vi "TankDrive.vi"   [LabVIEW 2011]
uses:
  <vilib>/Rock Robotics/WPI/Solenoid/Deprecated/WPI_SolenoidSetBool.vi
types:
  T1 = typedef "WPI_SolenoidDevRef.ctl" = cluster{"DevStatus":errorcluster, "Solenoid Module":T2, "Forward Solenoid Channel":T3, "Reverse Solenoid Channel":T3}
  T2 = typedef "FPGA_TypedefSolenoidModule.ctl" = enum16{"Solenoid Module 1", "Solenoid Module 2"}
  T3 = typedef "WPI_SolenoidChannel.ctl" = enum8{"Solenoid 1", "Solenoid 2", "Solenoid 3", "Solenoid 4", "Solenoid 5", "Solenoid 6", "Solenoid 7", "Solenoid 8", "Invalid"}
  T4 = typedef "WPI_JoystickDevRef.ctl" = cluster{"Device":T5}
  T5 = typedef "WPI_JoystickDeviceEnum.ctl" = enum16{"USB 1", "USB 2", "USB 3", "USB 4", "Kinect 1", "Kinect 2"}
  T6 = typedef "WPI_RobotDriveDevRef.ctl" = cluster{"DevStatus":errorcluster, "Motors[]":T7[], "Square Inputs":bool, "Max Output":dbl, "Isochronous":bool}
  T7 = typedef "WPI_MotorControlDeviceRef.ctl" = cluster{"DeviceStatus":errorcluster, "Type":enum16{"PWM", "CAN"}, "PWM":cluster{"Digital Module":T8, "PWM Channel":T9, "DeadBand":T10}, "CAN":cluster{"Device Number":u8, "Control Mode":T11, "Semaphore":T12, "Max Vout":dbl}, "Invert":bool, "TransformRef":T13, "InvTransformRef":T13}
  T8 = typedef "FPGA_TypedefDigitalModule.ctl" = enum16{"Digital Module 1", "Digital Module 2"}
  T9 = typedef "FPGA_DIOPWMChannel.ctl" = enum8{"PWM 1", "PWM 2", "PWM 3", "PWM 4", "PWM 5", "PWM 6", "PWM 7", "PWM 8", "PWM 9", "PWM 10", "Invalid"}
  T10 = typedef "WPI_PWMDeadband.ctl" = cluster{"Name":string, "maxPositivePwm":i32, "minPositivePwm":i32, "centerPwm":i32, "maxNegativePwm":i32, "minNegativePwm":i32, "angularRange":u16}
  T11 = typedef "WPI_CANJaguar_ControlMode.ctl" = enum8{"Percent VBus", "Current", "Speed", "Position", "Voltage"}
  T12 = typedef "Semaphore RefNum" = refnum<k1>
  T13 = typedef "WPI_PWMTransform_ConPane.ctl" = refnum<vi>
  T14 = typedef "WPI_JoystickButtonState.ctl" = cluster{"Button 1":bool, "Button 2":bool, "Button 3":bool, "Button 4":bool, "Button 5":bool, "Button 6":bool, "Button 7":bool, "Button 8":bool, "Button 9":bool, "Button 10":bool, "Button 11":bool, "Button 12":bool}
  T15 = cluster{"axis 1 (x)":dbl, "axis 2 (y)":dbl, "axis 3 (throttle)":dbl, "axis 4":dbl, "axis 5":dbl, "axis 6":dbl}
  T16 = typedef "WPI_DigitalOutputDevRef.ctl" = cluster{"Digital Module":T8, "DIO Channel":T17, "DevStatus":errorcluster}
  T17 = typedef "FPGA_DIOChannel.ctl" = enum8{"DIO 1", "DIO 2", "DIO 3", "DIO 4", "DIO 5", "DIO 6", "DIO 7", "DIO 8", "DIO 9", "DIO 10", "DIO 11", "DIO 12", "DIO 13", "DIO 14", "Invalid"}
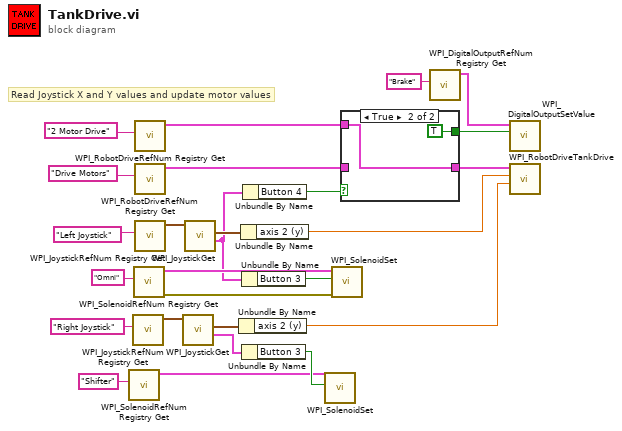
[diagram p0: block diagram]
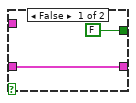
[diagram p2: hidden frame]
diagram:
  # "Read Joystick X and Y values and update motor values"
  n1 = call <vilib>:"WPI_SolenoidRefNum Registry Get.vi"("refnum name"="Shifter") -> ("SolenoidDevRef"=w24:T1)  [unwired: 1 in, 9 out]
  n2 = call <vilib>:"WPI_JoystickRefNum Registry Get.vi"("refnum name"="Right Joystick") -> ("JoystickDevRef"=w21:T4)  [unwired: 1 in, 9 out]
  n3 = call <vilib>:"WPI_SolenoidRefNum Registry Get.vi"("refnum name"="Omni") -> ("error out"=w11:errorcluster, "SolenoidDevRef"=w12:T1)  [unwired: 9 in]
  n4 = call <vilib>:"WPI_RobotDriveRefNum Registry Get.vi"("refnum name"="2 Motor Drive") -> ("RobotDriveDevRef"=w7:T6)  [unwired: 1 in, 9 out]
  n5 = call <vilib>:"WPI_RobotDriveRefNum Registry Get.vi"("refnum name"="Drive Motors") -> ("RobotDriveDevRef"=w4:T6)  [unwired: 1 in, 9 out]
  n6 = call <vilib>:"WPI_JoystickRefNum Registry Get.vi"("refnum name"="Left Joystick") -> ("JoystickDevRef"=w18:T4)  [unwired: 1 in, 9 out]
  n7 = call <vilib>:"WPI_JoystickGet.vi"("JoystickDevRef"=w21) -> ("Buttons"=w23:T14, "Axes"=w19:T15)  [unwired: 1 in, 4 out]
  n8 = call <vilib>:"WPI_JoystickGet.vi"("JoystickDevRef"=w18) -> ("Buttons"=w8:T14, "Axes"=w16:T15)  [unwired: 1 in, 4 out]
  n9 = Unbundle By Name(w19) -> ("axis 2 (y)"=w22:dbl)
  n10 = Unbundle By Name(w16) -> ("axis 2 (y)"=w15:dbl)
  n11 = Unbundle By Name(w8) -> ("Button 3"=w10:bool)
  n12 = Unbundle By Name(w23) -> ("Button 3"=w26:bool)
  n13 = Unbundle By Name(w8) -> ("Button 4"=w5:bool)
  n14 = call-poly <vilib>:"WPI_SolenoidSet.vi"("Value"=w26, "SolenoidDevRef"=w24) -> ()  [unwired: 1 in, 9 out]
  n15 = call-poly <vilib>:"WPI_SolenoidSet.vi"("error in (no error)"=w11, "Value"=w10, "SolenoidDevRef"=w12) -> ()  [unwired: 7 in, 2 out]
  n16 = case shown="True" w5 {
    tunnel: w7 -> [_ w30]
    tunnel: [w28 w30] -> w6
    tunnel: w4 -> [w28 _]
    tunnel: [FALSE ("Value") TRUE ("Value")] -> w1
    frame False {
    }
    frame True {
    }
  }
  n17 = call <vilib>:"WPI_DigitalOutputRefNum Registry Get.vi"("refnum name"="Brake") -> ("DigitalOutputDevRef"=w2:T16)  [unwired: 9 in, 1 out]
  n18 = call <vilib>:"WPI_DigitalOutputSetValue.vi"("Value"=w1, "DigitalOutputDevRef"=w2) -> ()  [unwired: 8 in, 2 out]
  n19 = call <vilib>:"WPI_RobotDriveTankDrive.vi"("Right axis value"=w22, "Left axis value"=w15, "RobotDriveDevRef"=w6) -> ()  [unwired: 7 in, 2 out]
